vi "Charger_Set Not Ready on Error.vi"(6 "Status Refnum":T1, 7 "error in":errorcluster) -> (0 "error out":errorcluster {"code" format="%.0x"}, 4 "ready status":bool)   [LabVIEW 2020]
uses:
  Charger_Status Refnum.ctl
  Drivers/Charger Test Set/Charger_Input Control.ctl
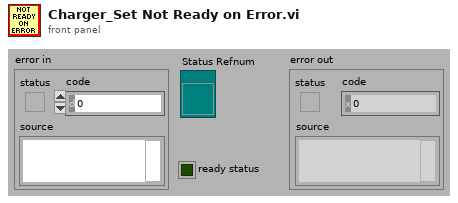
[diagram p1: front panel]
types:
  T1 = typedef "Charger_Status Refnum.ctl" = refnum<vi>
  T2 = typedef "Charger_Input Control.ctl" = cluster{"address":refnum<visa-resource-name>, "position":i32, "setpoint":dbl}
  T3 = cluster{"MICS ID":u32, "VBAT":dbl, "ChargingState":string, "VBAT Slide":dbl, "Status":string, "TemperatureLevel":dbl, "IPG_ReceivedLevel":dbl, "VBAT Target":dbl, "Charger Setpoint":dbl, "Index":i32, "Ready":bool, "Charger Inputs":T2, "MICS Inputs":cluster{"address":refnum<visa-resource-name>, "chan":u16, "ID":u32}}
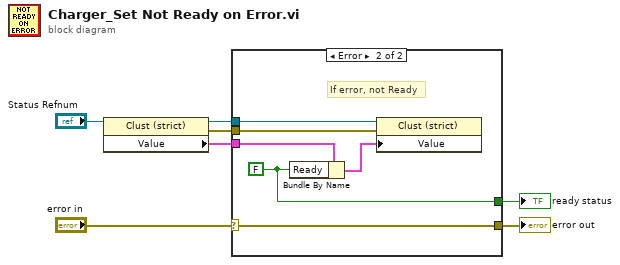
[diagram p0: block diagram]
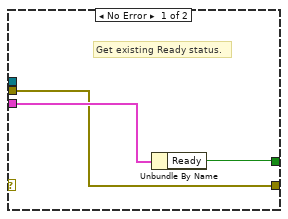
[diagram p2: hidden frame]
diagram:
  n1 = property class="Clust (strict)"(reference="Status Refnum") -> (reference out=w5:T1, error out=w6:errorcluster, "Value"=w4:T3)  [unwired: 1 in]
  n2 = case shown="Error" "error in" {
    selector: "error in" -> [_ w12]
    tunnel: w6 -> [w8 w16]
    tunnel: w5 -> [_ w15]
    tunnel: w4 -> [w9 w14]
    tunnel: [w8 w12] -> w2
    tunnel: [w10 w11] -> w1
    frame No Error {
      # "Get existing Ready status."
      n3 = Unbundle By Name(w9) -> ("Ready"=w10:bool)
    }
    frame Error {
      w11 = FALSE ("Ready")
      # "If error, not Ready"
      n4 = Bundle By Name(cluster=w14, "Ready"=w11) -> (w13:T3)
      n5 = property class="Clust (strict)"(reference=w15, error in=w16, "Value"=w13) -> ()  [unwired: 2 out]
    }
  }
  "error out" <- w2
  "ready status" <- w1
